vi "AMI1700_getinfo.vi"(8 "error in (no error)":errorcluster, 10 "string":string, 11 "VISA resource name":refnum<visa-resource-name>) -> (0 "error out":errorcluster, 2 "read buffer":string, 3 "VISA resource name 2":refnum<visa-resource-name>)   [LabVIEW 2019]
uses:
  <vilib>/Instr/_visa.llb/VISA Configure Serial Port (Instr).vi
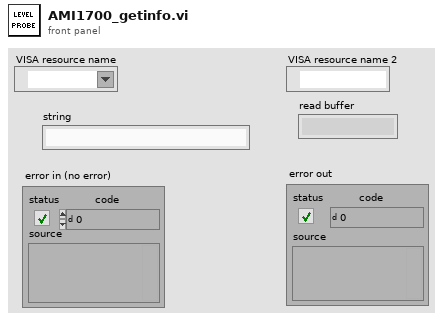
[diagram p1: front panel]
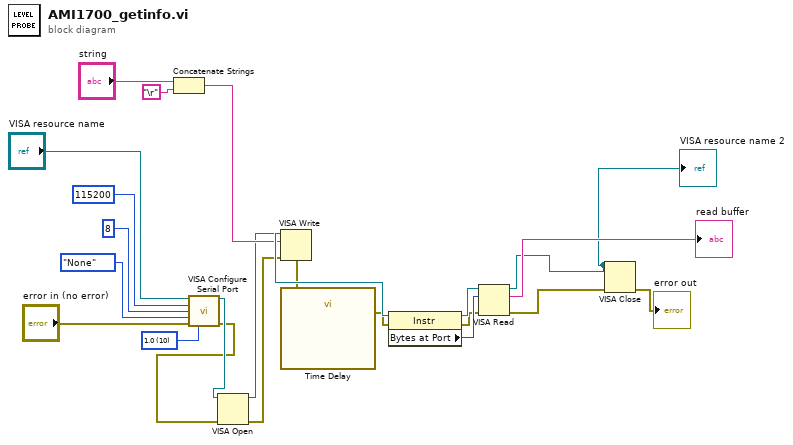
[diagram p0: block diagram]
diagram:
  w17 = u16 10 items=["1.0"=10, "1.5"=15, "2.0"=20] ("stop bits (10: 1 bit)")
  n1 = Concatenate Strings("string", "\r") -> (w14:string)
  n2 = call-poly "VISA Configure Serial Port"("VISA resource name"="VISA resource name", "baud rate (9600)"=u32 115200, "data bits (8)"=u16 8, "parity (0:none)"=enum16{"None", "Odd", "Even", "Mark", "Space"}."None", "error in (no error)"="error in (no error)", "stop bits (10: 1 bit)"=w17) -> ("VISA resource name out"=w7:refnum<visa-resource-name>, "error out"=w5:errorcluster)  [unwired: 8 in]
  n3 = VISA Open(error in (no error)=w5, VISA resource name=w7) -> (VISA resource name=w6:refnum<visa-resource-name>, error out=w4:errorcluster)  [unwired: 3 in]
  n4 = VISA Write(VISA resource name=w6, write buffer=w14, error in (no error)=w4) -> (VISA resource name out=w23:refnum<visa-resource-name>, error out=w10:errorcluster)  [unwired: 1 out]
  n5 = call "Time Delay"("error in (no error)"=w10) -> ("error out"=w9:errorcluster)  [unwired: 10 in]
  n6 = property class="Instr"(reference=w23, error in=w9) -> (reference out=w22:refnum<visa-resource-name>, error out=w11:errorcluster, "Bytes at Port"=w13:u32)
  n7 = VISA Read(VISA resource name=w22, byte count=w13, error in (no error)=w11) -> (VISA resource name out=w1:refnum<visa-resource-name>, read buffer=→"read buffer":string, error out=w2:errorcluster)  [unwired: 1 out]
  "VISA resource name 2" <- w1
  n8 = VISA Close(VISA resource name=w1, error in (no error)=w2) -> (error out=→"error out":errorcluster)
